vi "Get Display Items.vi"(8 "error in (no error)":errorcluster, 11 "Preview in":refnum<class "Preview.lvclass">) -> (0 "error out":errorcluster, 1 "Scalar Items":T1, 2 "Wfm Items":T2, 3 "Preview out":refnum<class "Preview.lvclass">)   [LabVIEW 2018, in "Preview Window.lvlib" / "Preview.lvclass"]
uses:
  Preview.lvclass
  Preview.lvclass/Preview.ctl
  Cfg Grandmaster/Class Chassis BOM/Chassis BOM.lvclass/Chassis BOM.ctl
  Cfg Grandmaster/Class Chassis BOM/Read Chassis Alias.vi
  Cfg Grandmaster/Class Timing Group/Read Rate.vi
  Cfg Grandmaster/Class Chassis Cfg/ChassisCfg.lvclass
  Cfg Grandmaster/Class Timing Group/TimingGrp.lvclass
  Cfg Grandmaster/Class Chan Group/ChanGrp.lvclass
  Cfg Grandmaster/Class Chassis BOM/Chassis BOM.lvclass
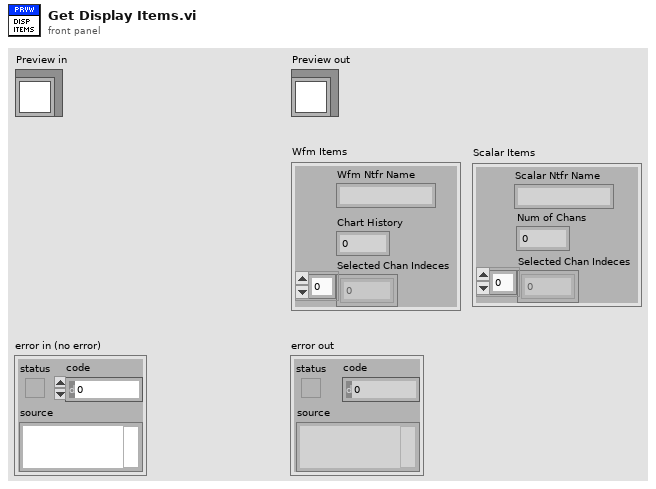
[diagram p1: front panel]
types:
  T1 = cluster{"Scalar Ntfr Name":string, "Num of Chans":i32, "Selected Chan Indeces":i32[]}
  T2 = cluster{"Wfm Ntfr Name":string, "Chart History":i32, "Selected Chan Indeces":i32[]}
  T3 = typedef "Selected Group.ctl" = cluster{"ChanGroup":i32, "Rate Class":T4}
  T4 = typedef "TE_Designator.ctl" = enum16{"High Speed", "Low Speed"}
  T5 = cluster{"Scalar Notifier":string, i32, "Selected Chan Indeces":i32[]}
  T6 = cluster{"Wfm Notifier":string, i32, "Selected Chan Indeces":i32[]}
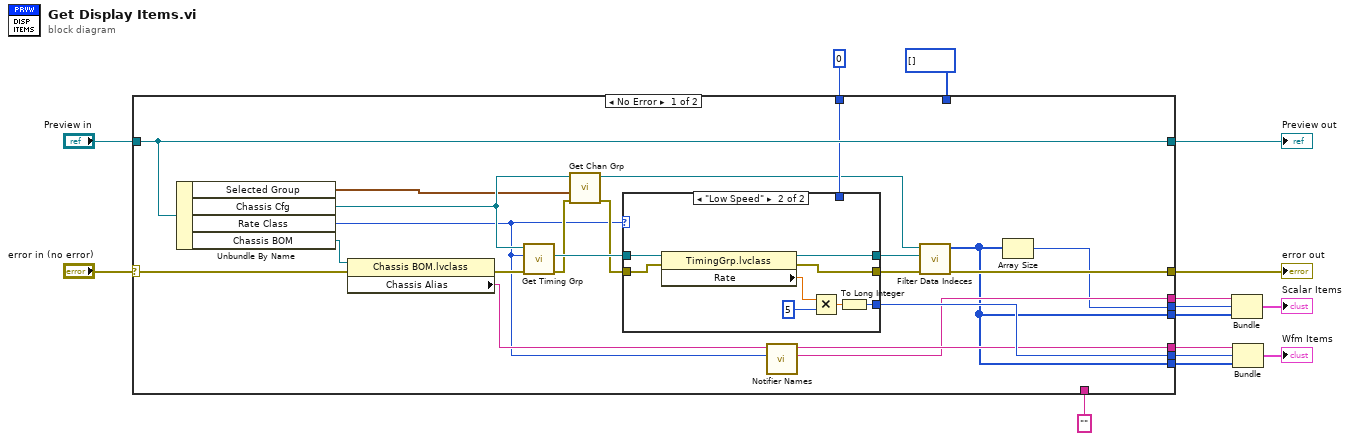
[diagram p0: block diagram]
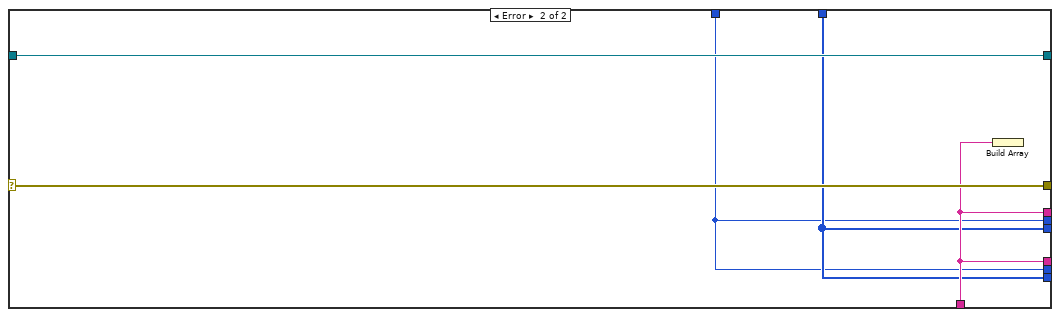
[diagram p3: hidden frame]
diagram:
  n1 = case shown="No Error" "error in (no error)" {
    selector: "error in (no error)" -> [w28 w52]
    tunnel: [w18 w52] -> w14
    tunnel: [w36 w51] -> w12
    tunnel: "Preview in" -> [w36 w51]
    tunnel: [w17 w49] -> w8
    tunnel: [w20 w50] -> w6
    tunnel: [w25 w48] -> w5
    tunnel: "" -> [_ w50]
    tunnel: i32[] [] ("Selected Chan Indeces") -> [_ w49]
    tunnel: 0 -> [w24 w48]
    tunnel: [w19 w50] -> w4
    tunnel: [w17 w49] -> w2
    tunnel: [w16 w48] -> w1
    frame No Error {
      n2 = Unbundle By Name(w36) -> ("Selected Group"=w31:T3, "Chassis Cfg"=w32:refnum<class "ChassisCfg.lvclass">, "Rate Class"=w21:T4, "Chassis BOM"=w26:refnum<class "Chassis BOM.lvclass">)
      n3 = property class="Chassis BOM.lvclass"(reference=w26, error in=w28) -> (error out=w27:errorcluster, "Chassis Alias"=w22:string)  [unwired: 1 out]
      n4 = call "Get Timing Grp.vi"("error in (no error)"=w27, "Timing Engine"=w21, "Chassis Cfg"=w32) -> ("error out"=w30:errorcluster, "Timing Groups"=w35:refnum<class "TimingGrp.lvclass">)  [unwired: 6 in, 1 out]
      n5 = call "Get Chan Grp.vi"("error in (no error)"=w30, "Selected Grp"=w31, "Chassis Cfg"=w32) -> ("error out"=w29:errorcluster, "Chan Group"=w23:refnum<class "ChanGrp.lvclass">)  [unwired: 7 in]
      n6 = case shown="\"Low Speed\"" w21 {
        tunnel: [w39 w43] -> w33
        tunnel: [w37 w45] -> w25
        tunnel: w35 -> [w39 w42]
        tunnel: w29 -> [w38 w41]
        tunnel: [w38 w40] -> w34
        tunnel: w24 -> [w37 _]
        frame "High Speed" {
        }
        frame "Low Speed" {
          n7 = property class="TimingGrp.lvclass"(reference=w42, error in=w41) -> (reference out=w43:refnum<class "TimingGrp.lvclass">, error out=w40:errorcluster, "Rate"=w44:dbl)
          n8 = Multiply(x=w44, y=5) -> (x*y=w46:dbl)
          n9 = To Long Integer(number=w46) -> (32bit integer=w45:i32)
        }
      }
      n10 = call "Notifier Names.vi"("TimingEngine"=w21, "Chassis Name"=w22) -> ("Scalar Notifier"=w19:string, "Wfm Notifier"=w20:string)  [unwired: 8 in]
      n11 = call "Filter Data Indeces.vi"("error in (no error)"=w34, "TimingGrp.lvclass"=w33, "Selected Group"=w23) -> ("error out"=w18:errorcluster, "Selected Chan Indeces"=w17:i32[])  [unwired: 6 in, 1 out]
      n12 = Array Size(array=w17) -> (size(s)=w16:i32)
    }
    frame Error {
      n13 = Build Array(w50) -> ()  [unwired: 1 out]
    }
  }
  "error out" <- w14
  "Preview out" <- w12
  n14 = Bundle("Scalar Notifier"=w4, w1, "Selected Chan Indeces"=w2) -> (→"Scalar Items":T5)  [unwired: 1 in]
  n15 = Bundle("Wfm Notifier"=w6, w5, "Selected Chan Indeces"=w8) -> (→"Wfm Items":T6)  [unwired: 1 in]
